vi "vislt_FGPA_Main_test 16.vi"() -> ()   [LabVIEW 2014]
panel:
  out "error out 2":errorcluster
  out "error out":errorcluster
  out "Boolean Indicator":bool
  out "FXP Indicator":fxp<+/-,16,16>
  out "I32 Indicator":i32
  out "SGL Indicator":sgl
  out "Boolean Control":bool
  in  "FXP Control":fxp<+/-,16,16>
  out "I32 Control":i32
  out "SGL Control":sgl
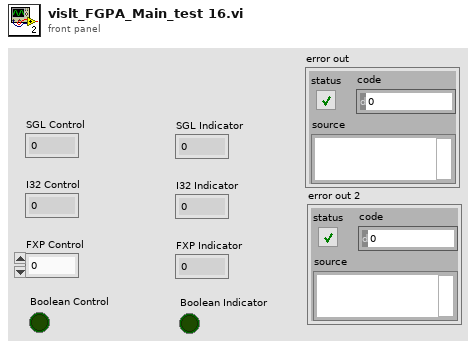
[diagram p1: front panel]
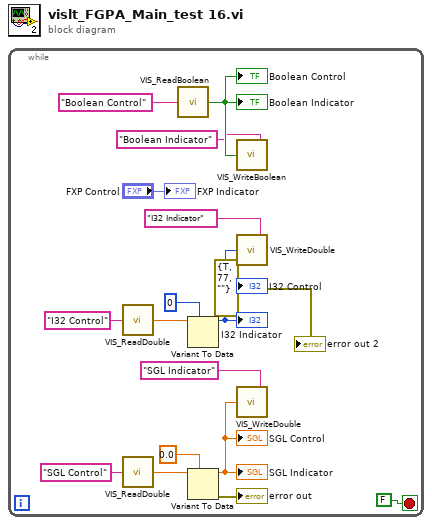
[diagram p0: block diagram]
diagram:
  n1 = while {
    stop <- FALSE stop-if-true
    n2 = call <nishared>:"VIS_ReadDouble.vi"("DataItem"="I32 Control") -> ("Data out"=w9:dbl)
    n3 = call <nishared>:"VIS_ReadDouble.vi"("DataItem"="SGL Control") -> ("Data out"=w13:dbl)
    n4 = call <nishared>:"VIS_ReadBoolean.vi"("DataItem"="Boolean Control") -> ("Data out"=w5:bool)
    "Boolean Control" <- w5
    "Boolean Indicator" <- w5
    n5 = Variant To Data(type=0 ("I32 Control"), Variant=w9) -> (data=w7:i32)  [unwired: 1 in, 1 out]
    "I32 Control" <- w7
    "I32 Indicator" <- w7
    n6 = Variant To Data(type=sgl 0.0 ("SGL Control"), Variant=w13) -> (data=w11:sgl, error out=→"error out":errorcluster)  [unwired: 1 in]
    "SGL Control" <- w11
    "SGL Indicator" <- w11
    n7 = call <nishared>:"VIS_WriteBoolean.vi"("DataItem"="Boolean Indicator", "Data in"=w5) -> ()
    n8 = call <nishared>:"VIS_WriteDouble.vi"("DataItem"="I32 Indicator", "Data in"=w7) -> ()
    n9 = call <nishared>:"VIS_WriteDouble.vi"("DataItem"="SGL Indicator", "Data in"=w11) -> ()
    "FXP Indicator" <- "FXP Control"
    "error out 2" <- errorcluster {"status"=TRUE, "code"=77, "source"=""} ("error out 2")
  }
